vi "Pump Status.vi"(0 "ASIA Pump C Settings in":T2, 11 "error in (no error)":errorcluster) -> (1 "pressure":dbl, 3 "PumpStatusCode":T1(ring)=enum."Idle", 4 "ASIA Pump C Settings out":T2, 6 "Pump On?":enum16{"Off", "On", "Not Initialized"}(ring), 8 "Overpressure":bool, 10 "Connection Error":bool, 12 "syringeSize (ml)":sgl, 14 "pumpRate":dbl format="%.2f", 15 "error out":errorcluster)   [LabVIEW 2018, in "ASIA Pump.lvlib"]
uses:
  ASIA Pump.lvlib
  Pump Settings.ctl
  Program Files (x86)/Pfizer/FAST/data/AsiaPumpInterface.dll
panel:
  out "error":string
  out "Task Completed":u8
  out "pumpIndex":i32
  out "Error":string
  out "lastOverPressure":i32
  out "errorCode":i32
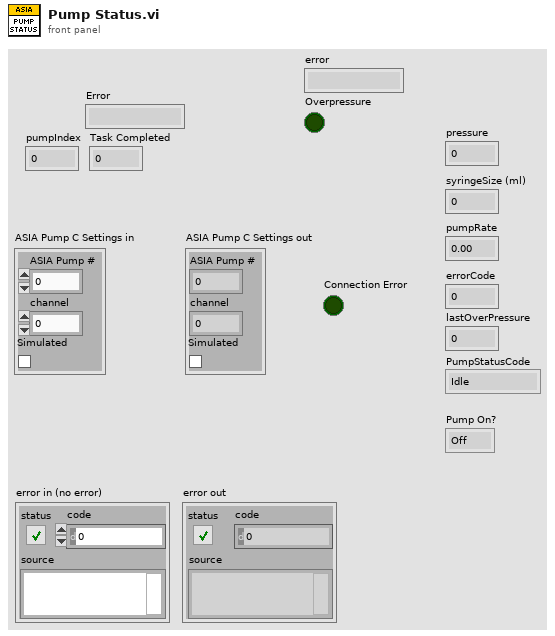
[diagram p1: front panel]
types:
  T1 = enum16{"Error", "Uninitialised", "Initialising", "Idle", "Filling", "Full", "Emptying", "Empty", "Pumping", "Default"}
  T2 = typedef "ASIA Pump.lvlib/Pump Settings.ctl" = cluster{"ASIA Pump #":i32, "channel":i32, "Simulated":bool}
  T3 = cluster{"Busy":bool, "PumpCnt":dbl, "RemoteEntered":bool, "OverpressureSet":bool}[]
  T4 = cluster{"Busy":bool, "PumpCnt":dbl, "RemoteEntered":bool, "OverpressureSet":bool}
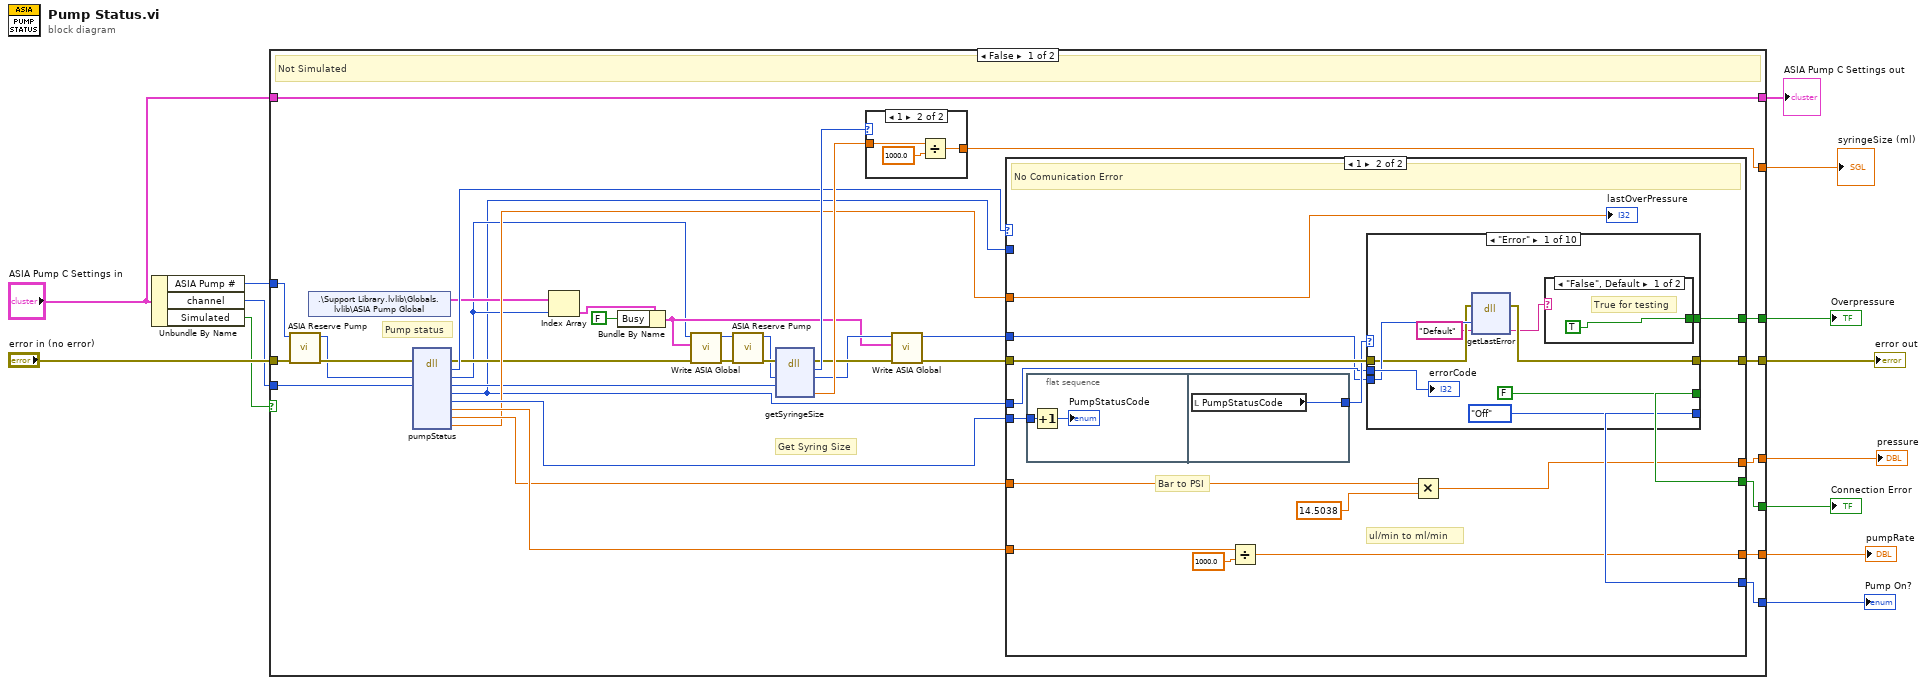
[diagram p0: block diagram]
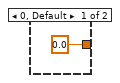
[diagram p2: hidden frame]
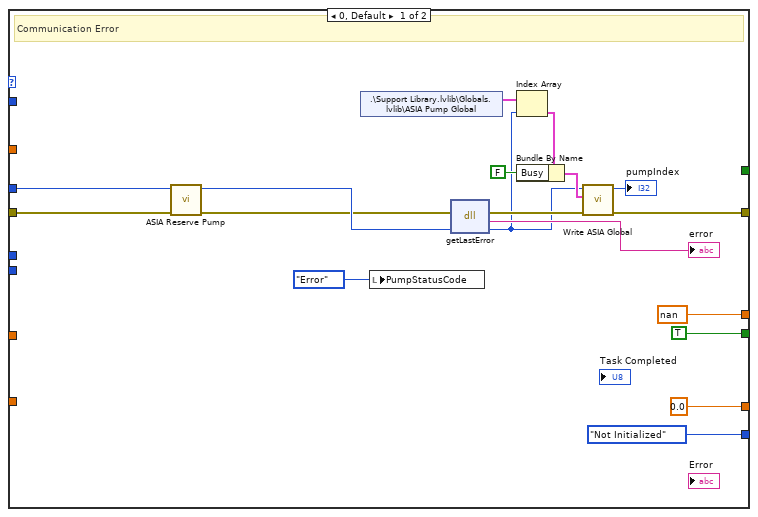
[diagram p3: hidden frame]
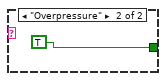
[diagram p4: hidden frame]
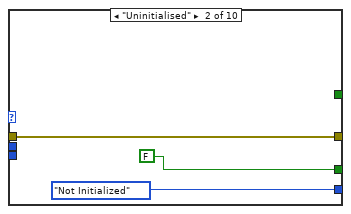
[diagram p5: hidden frame]
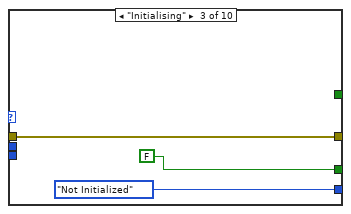
[diagram p6: hidden frame]
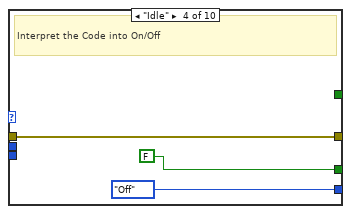
[diagram p7: hidden frame]
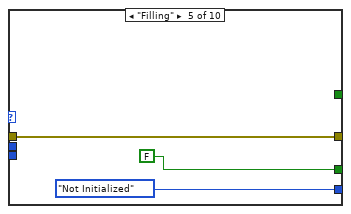
[diagram p8: hidden frame]
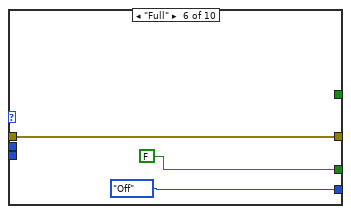
[diagram p9: hidden frame]
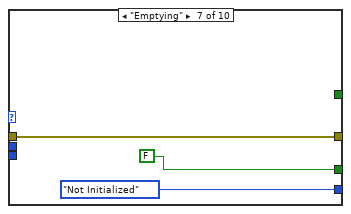
[diagram p10: hidden frame]
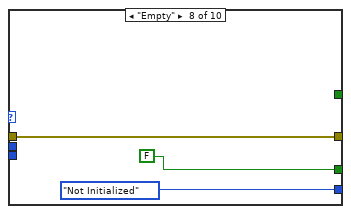
[diagram p11: hidden frame]
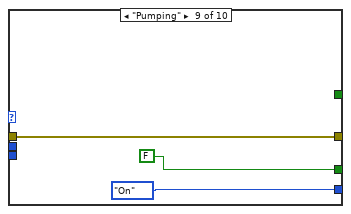
[diagram p12: hidden frame]
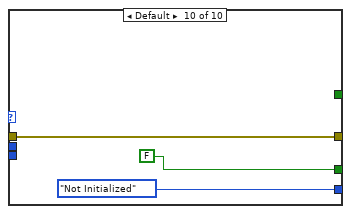
[diagram p13: hidden frame]
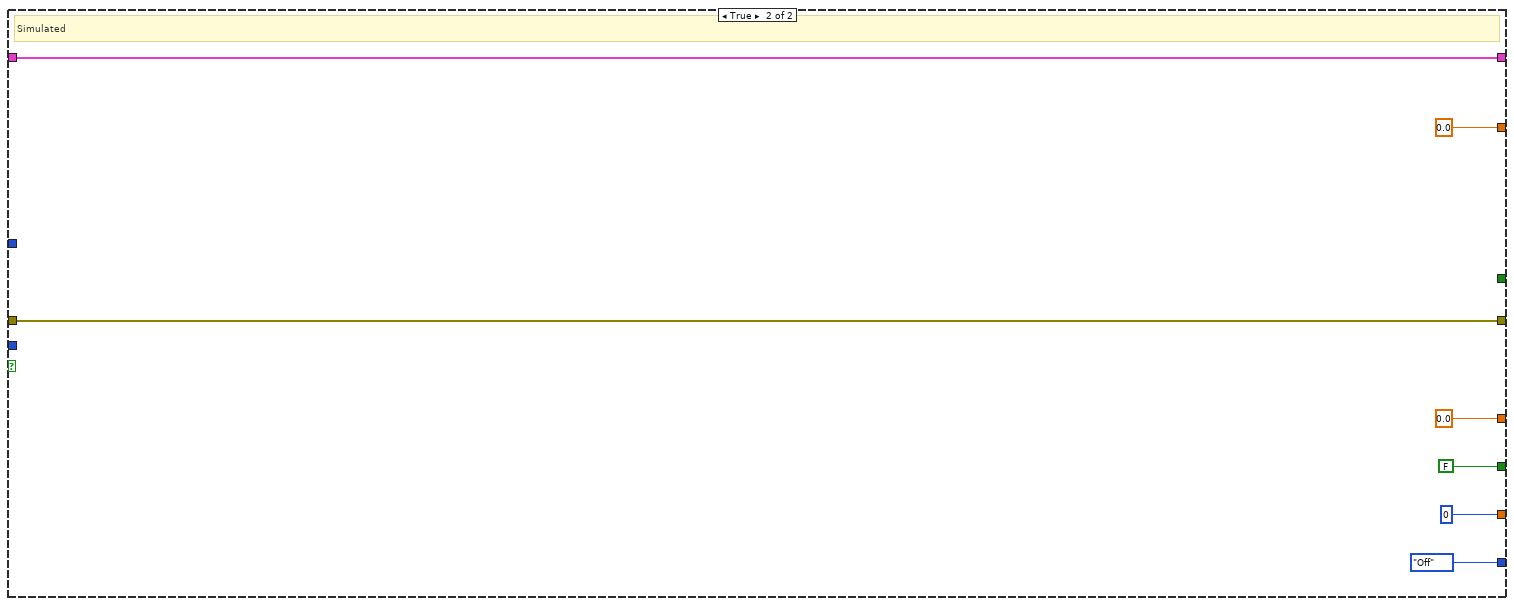
[diagram p14: hidden frame]
diagram:
  n1 = Unbundle By Name("ASIA Pump C Settings in") -> ("ASIA Pump #"=w2:i32, "channel"=w1:i32, "Simulated"=w3:bool)
  n2 = case shown="False" w3 {
    tunnel: [w49 FALSE ("Connection Error")] -> w13
    tunnel: [w48 w129] -> w12
    tunnel: [w47 0 ("pumpRate")] -> w11
    tunnel: [w46 enum16{"Off", "On", "Not Initialized"}."Off" ("Pump On?")] -> w10
    tunnel: [w41 sgl 0.0 ("syringeSize")] -> w9
    tunnel: [w43 sgl 0.0 ("pressure")] -> w8
    tunnel: "ASIA Pump C Settings in" -> [w42 w130]
    tunnel: [w42 w130] -> w6
    tunnel: "error in (no error)" -> [w33 w129]
    tunnel: w2 -> [w31 _]
    tunnel: w1 -> [w40 _]
    tunnel: [w14 _] -> w4
    frame False {
      # "Get Syring Size"
      # "Pump status"
      # "Not Simulated"
      n3 = call "ASIA Reserve Pump.vi"("error in (no error)"=w33, "ASIA Pump #"=w31) -> ("error out"=w32:errorcluster, "ASIA Pump #"=w30:i32)  [unwired: 8 in]
      n4 = shared-variable ".\\Support Library.lvlib\\Globals.lvlib\\ASIA Pump Global"() -> (w18:T3)  [unwired: 1 in, 1 out]
      n5 = dll-call lib="C:/Program Files (x86)/Pfizer/FAST/data/AsiaPumpInterface.dll" fn="pumpStatus"(error in=w32, "pumpNum"=w30, "channel"=w40) -> (error out=w29:errorcluster, "Task Completed"=w39:u8, "pumpNum"=w16:u32, "channel"=w34:u32, "errorCode"=w15:i32, "pumpState"=w38:i32, "pumpRate"=w37:sgl, "pressure"=w36:sgl, "lastOverPressure"=w35:sgl)  [unwired: 7 in, 1 out]
      n6 = Index Array(array=w18, index=w16) -> (element=w17:T4)
      n7 = Bundle By Name(cluster=w17, "Busy"=FALSE) -> (w19:T4)
      n8 = call "Write ASIA Global.vi"("error in (no error)"=w29, "ASIA Global"=w19, "Pump Number"=w16) -> ("error out"=w27:errorcluster, "Pump Number"=w26:i32)  [unwired: 7 in]
      n9 = call "ASIA Reserve Pump.vi"("error in (no error)"=w27, "ASIA Pump #"=w26) -> ("error out"=w28:errorcluster, "ASIA Pump #"=w25:i32)  [unwired: 8 in]
      n10 = dll-call lib="C:/Program Files (x86)/Pfizer/FAST/data/AsiaPumpInterface.dll" fn="getSyringeSize"(error in=w28, "pumpNum"=w25, "channel"=w34) -> (error out=w24:errorcluster, "Task Completed"=w45:u8, "pumpNum"=w22:u32, "syringeSize"=w44:sgl)  [unwired: 4 in, 1 out]
      n11 = case shown="1" w45 {
        tunnel: w44 -> [_ w52]
        tunnel: [sgl 0.0 ("syringeSize") w51] -> w41
        frame 0, Default {
        }
        frame 1 {
          n12 = Divide(x=w52, y=1000.0) -> (x/y=w51:dbl)
        }
      }
      n13 = call "Write ASIA Global.vi"("error in (no error)"=w24, "ASIA Global"=w19, "Pump Number"=w22) -> ("error out"=w23:errorcluster, "Pump Number"=w21:i32)  [unwired: 7 in]
      n14 = case shown="1" w39 {
        tunnel: [TRUE w87] -> w49
        tunnel: [w59 w86] -> w48
        tunnel: w23 -> [w65 w85]
        tunnel: w37 -> [_ w76]
        tunnel: w38 -> [_ w83]
        tunnel: w15 -> [_ _]
        tunnel: w36 -> [_ w79]
        tunnel: w35 -> [_ w84]
        tunnel: [0.0 ("pumpRate") w75] -> w47
        tunnel: [enum16{"Off", "On", "Not Initialized"}."Not Initialized" ("Pump On?") w81] -> w46
        tunnel: [sgl nan ("pressure") w78] -> w43
        tunnel: w21 -> [w64 w73]
        tunnel: w15 -> [_ w74]
        tunnel: [_ w72] -> w14
        frame 0, Default {
          # "Communication Error"
          n15 = call "ASIA Reserve Pump.vi"("error in (no error)"=w65, "ASIA Pump #"=w64) -> ("error out"=w62:errorcluster, "ASIA Pump #"=w63:i32)  [unwired: 8 in]
          n16 = shared-variable ".\\Support Library.lvlib\\Globals.lvlib\\ASIA Pump Global"() -> (w56:T3)  [unwired: 1 in, 1 out]
          n17 = local write "PumpStatusCode"(T1."Error" ("PumpStatusCode")) -> ()
          n18 = dll-call lib="C:/Program Files (x86)/Pfizer/FAST/data/AsiaPumpInterface.dll" fn="getLastError"(error in=w62, "pumpIndex"=w63) -> (error out=w61:errorcluster, "error"=→"error":string, "pumpIndex"=w54:i32)  [unwired: 2 in, 1 out]
          n19 = Index Array(array=w56, index=w54) -> (element=w55:T4)
          n20 = Bundle By Name(cluster=w55, "Busy"=FALSE) -> (w57:T4)
          n21 = call "Write ASIA Global.vi"("error in (no error)"=w61, "ASIA Global"=w57, "Pump Number"=w54) -> ("error out"=w59:errorcluster, "Pump Number"=→"pumpIndex":i32)  [unwired: 7 in]
        }
        frame 1 {
          # "ul/min to ml/min"
          # "Bar to PSI"
          # "No Comunication Error"
          n22 = flat-sequence {
            tunnel: w83 -> [w89]
            tunnel: [w90] -> w82
            frame #0 {
              n23 = Increment(x=w89) -> (x+1=→"PumpStatusCode":i32)
            }
            frame #1 {
              n24 = local read "PumpStatusCode"() -> (w90:T1)
            }
          }
          n25 = Divide(x=w76, y=1000.0) -> (x/y=w75:dbl)
          n26 = case shown="\"Error\"" w82 {
            tunnel: [FALSE FALSE FALSE FALSE FALSE FALSE FALSE FALSE FALSE FALSE] -> w87
            tunnel: w85 -> [w95 w103 w106 w109 w112 w115 w118 w121 w124 w127]
            tunnel: [w94 w103 w106 w109 w112 w115 w118 w121 w124 w127] -> w86
            tunnel: w73 -> [w96 _ _ _ _ _ _ _ _ _]
            tunnel: [enum16{"Off", "On", "Not Initialized"}."Off" ("Pump On?") enum16{"Off", "On", "Not Initialized"}."Not Initialized" ("Pump On?") enum16{"Off", "On", "Not Initialized"}."Not Initialized" ("Pump On?") enum16{"Off", "On", "Not Initialized"}."Off" ("Pump On?") enum16{"Off", "On", "Not Initialized"}."Not Initialized" ("Pump On?") enum16{"Off", "On", "Not Initialized"}."Off" ("Pump On?") enum16{"Off", "On", "Not Initialized"}."Not Initialized" ("Pump On?") enum16{"Off", "On", "Not Initialized"}."Not Initialized" ("Pump On?") enum16{"Off", "On", "Not Initialized"}."On" ("Pump On?") enum16{"Off", "On", "Not Initialized"}."Not Initialized" ("Pump On?")] -> w81
            tunnel: w74 -> [w97 _ _ _ _ _ _ _ _ _]
            tunnel: [w91 _ _ _ _ _ _ _ _ _] -> w72
            frame "Error" {
              n27 = dll-call lib="C:/Program Files (x86)/Pfizer/FAST/data/AsiaPumpInterface.dll" fn="getLastError"(error in=w95, "pumpNum"=w96, "Error"="Default") -> (error out=w94:errorcluster, "Error"=w92:string)  [unwired: 4 in, 1 out]
              n28 = case shown="\"False\", Default" w92 {
                tunnel: [TRUE ("Overpressure") TRUE ("Overpressure")] -> w91
                frame "False", Default {
                  # "True for testing"
                }
                frame "Overpressure" {
                }
              }
              "errorCode" <- w97
            }
            frame "Uninitialised" {
            }
            frame "Initialising" {
            }
            frame "Idle" {
              # "Interpret the Code into On/Off"
            }
            frame "Filling" {
            }
            frame "Full" {
            }
            frame "Emptying" {
            }
            frame "Empty" {
            }
            frame "Pumping" {
            }
            frame Default {
            }
          }
          n29 = Multiply(x=w79, y=14.5038) -> (x*y=w78:dbl)
          "lastOverPressure" <- w84
        }
      }
    }
    frame True {
      # "Simulated"
    }
  }
  "error out" <- w12
  "ASIA Pump C Settings out" <- w6
  "Connection Error" <- w13
  "pumpRate" <- w11
  "Pump On?" <- w10
  "syringeSize (ml)" <- w9
  "pressure" <- w8
  "Overpressure" <- w4
